vi "sendMessage.vi"(6 "Message (\"\" => closes the window)":string, 8 "error in (no error)":errorcluster, 11 "guiTemplates in":refnum<class "stillnessHelper.lvclass">) -> (0 "error out":errorcluster, 3 "guiTemplates out":refnum<class "stillnessHelper.lvclass">)   [LabVIEW 2022 SP3, in "stillnessHelper.lvclass"]
uses:
  stillnessHelper.lvclass
  stillnessHelper.lvclass/stillnessHelper.ctl
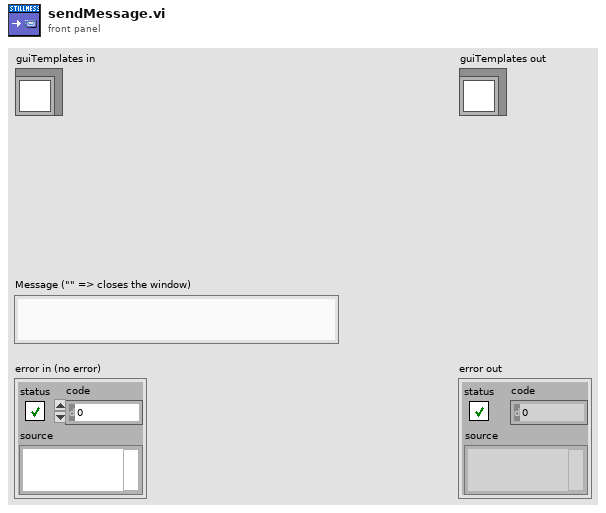
[diagram p1: front panel]
types:
  T1 = enum32{"Invalid", "Standard", "Closed", "Hidden", "Minimized", "Maximized"}
  T2 = typedef "LVRectTypeDef.ctl" = cluster{"Left":i16, "Top":i16, "Right":i16, "Bottom":i16}
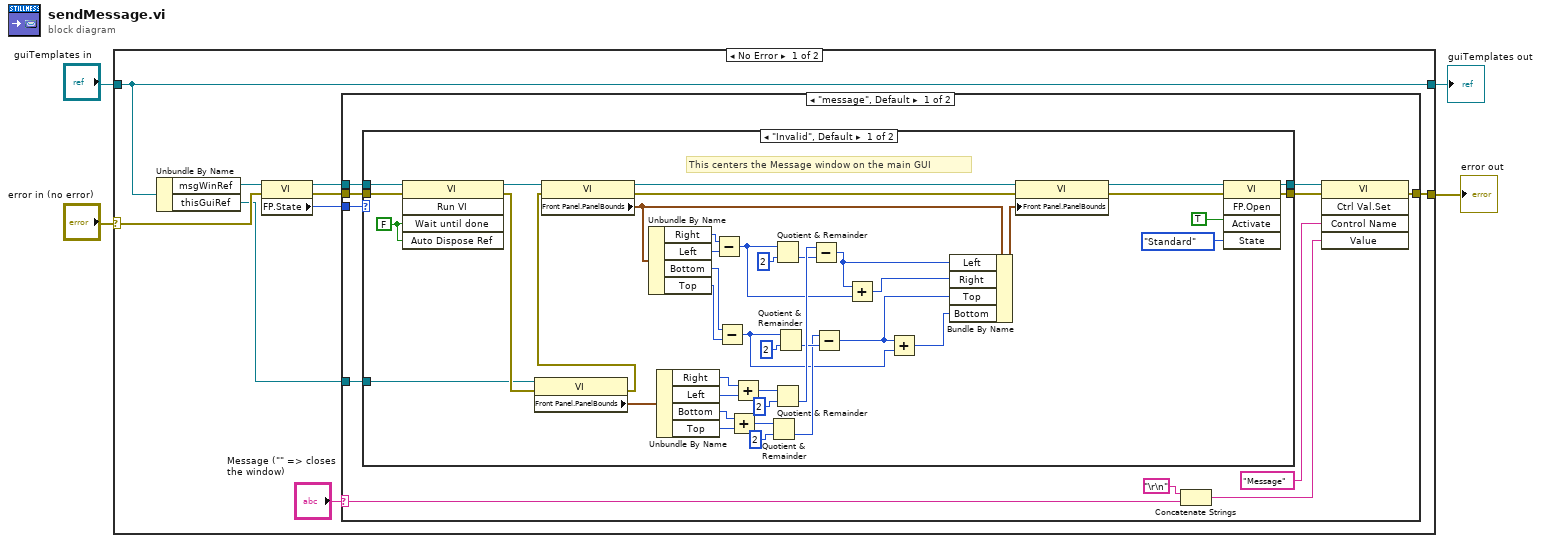
[diagram p0: block diagram]
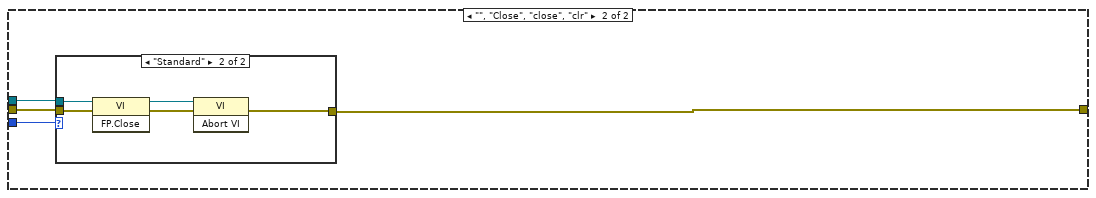
[diagram p3: hidden frame]
diagram:
  n1 = case shown="No Error" "error in (no error)" {
    selector: "error in (no error)" -> [w9 w80]
    tunnel: [w11 w80] -> w3
    tunnel: [w13 w79] -> w1
    tunnel: "guiTemplates in" -> [w13 w79]
    frame No Error {
      n2 = Unbundle By Name(w13) -> ("msgWinRef"=w10:refnum<vi>, "thisGuiRef"=w5:refnum<vi>)
      n3 = property class="VI"(reference=w10, error in=w9) -> (reference out=w8:refnum<vi>, error out=w7:errorcluster, "FP.State"=w6:T1)
      n4 = case shown="\"message\", Default" "Message (\"\" => closes the window)" {
        selector: "Message (\"\" => closes the window)" -> [w15 _]
        tunnel: [w18 w72] -> w11
        tunnel: w8 -> [w22 w71]
        tunnel: w7 -> [w23 w70]
        tunnel: w6 -> [w24 w69]
        tunnel: w5 -> [w21 _]
        frame "message", Default {
          n5 = case shown="\"Invalid\", Default" w24 {
            tunnel: [w56 w68] -> w19
            tunnel: w23 -> [w64 w68]
            tunnel: w22 -> [w65 w67]
            tunnel: w21 -> [w62 _]
            tunnel: [w55 w67] -> w17
            frame "Invalid", Default {
              w66 = FALSE ("Wait Until Done")
              # "This centers the Message window on the main GUI"
              n6 = invoke class="VI" method="Run VI"(reference=w65, error in=w64, "Wait until done"=w66, "Auto Dispose Ref"=w66) -> (reference out=w57:refnum<vi>, error out=w63:errorcluster)  [unwired: 1 in, 3 out]
              n7 = property class="VI"(reference=w62, error in=w63) -> (error out=w26:errorcluster, "Front Panel.PanelBounds"=w25:T2)  [unwired: 1 out]
              n8 = property class="VI"(reference=w57, error in=w26) -> (reference out=w49:refnum<vi>, error out=w48:errorcluster, "Front Panel.PanelBounds"=w50:T2)
              n9 = Unbundle By Name(w50) -> ("Right"=w52:i16, "Left"=w51:i16, "Bottom"=w32:i16, "Top"=w31:i16)
              n10 = Unbundle By Name(w25) -> ("Right"=w41:i16, "Left"=w42:i16, "Bottom"=w36:i16, "Top"=w35:i16)
              n11 = Subtract(x=w52, y=w51) -> (x-y=w46:i16)
              n12 = Subtract(x=w32, y=w31) -> (x-y=w28:i16)
              n13 = Add(x=w36, y=w35) -> (x+y=w38:i16)
              n14 = Add(x=w41, y=w42) -> (x+y=w37:i16)
              n15 = Quotient & Remainder(x=w38, y=i16 2) -> (floor(x/y)=w30:i16)  [unwired: 1 out]
              n16 = Quotient & Remainder(x=w46, y=i16 2) -> (floor(x/y)=w44:i16)  [unwired: 1 out]
              n17 = Quotient & Remainder(x=w37, y=i16 2) -> (floor(x/y)=w54:i16)  [unwired: 1 out]
              n18 = Quotient & Remainder(x=w28, y=i16 2) -> (floor(x/y)=w34:i16)  [unwired: 1 out]
              n19 = Subtract(x=w54, y=w44) -> (x-y=w43:i16)
              n20 = Subtract(x=w30, y=w34) -> (x-y=w29:i16)
              n21 = Add(x=w43, y=w46) -> (x+y=w45:i16)
              n22 = Add(x=w29, y=w28) -> (x+y=w27:i16)
              n23 = Bundle By Name(cluster=w50, "Left"=w43, "Right"=w45, "Top"=w29, "Bottom"=w27) -> (w47:T2)
              n24 = property class="VI"(reference=w49, error in=w48, "Front Panel.PanelBounds"=w47) -> (reference out=w60:refnum<vi>, error out=w61:errorcluster)
              n25 = invoke class="VI" method="FP.Open"(reference=w60, error in=w61, "Activate"=TRUE, "State"=T1."Standard") -> (reference out=w55:refnum<vi>, error out=w56:errorcluster)  [unwired: 1 in, 3 out]
            }
            frame "Standard" {
            }
          }
          n26 = Concatenate Strings("\r\n", w15) -> (w14:string)
          n27 = invoke class="VI" method="Ctrl Val.Set"(reference=w17, error in=w19, "Control Name"="Message", "Value"=w14) -> (error out=w18:errorcluster)  [unwired: 1 in, 4 out]
        }
        frame "", "Close", "close", "clr" {
          n28 = case shown="\"Standard\"" w69 {
            tunnel: [w73 w74] -> w72
            tunnel: w70 -> [w73 w77]
            tunnel: w71 -> [_ w78]
            frame "Invalid", Default {
            }
            frame "Standard" {
              n29 = invoke class="VI" method="FP.Close"(reference=w78, error in=w77) -> (reference out=w76:refnum<vi>, error out=w75:errorcluster)  [unwired: 1 in, 1 out]
              n30 = invoke class="VI" method="Abort VI"(reference=w76, error in=w75) -> (error out=w74:errorcluster)  [unwired: 1 in, 2 out]
            }
          }
        }
      }
    }
    frame Error {
    }
  }
  "error out" <- w3
  "guiTemplates out" <- w1
